vi "Init Hardware.vi"(8 "error in (no error)":errorcluster, 11 "Keithley in":refnum<class "Keithley Driver.lvclass">) -> (0 "error out":errorcluster, 3 "Keithley out":refnum<class "Keithley Driver.lvclass">)   [LabVIEW 2016, in "Keithley Driver.lvclass"]
uses:
  Keithley Driver.lvclass
  C:/github/NHMFL_Core/Libraries/Instruments/Instrument Driver/Instrument Driver.lvclass
  C:/github/NHMFL_Core/Libraries/Instruments/VISA Instrument/VISA Instrument.lvclass
  Instrument Driver/Instrument Driver.lvclass/Instrument Driver.ctl
  VISA Instrument/VISA Instrument.lvclass/VISA Instrument.ctl
  Instrument Driver/Read Recorder name.vi
  VISA Instrument/Read VISA resource.vi
  Instrument Driver/Write Channel names.vi
  Instrument Driver/Write Channel units.vi
  VISA Instrument/Write VISA resource.vi
  Read Keithley user configuration.vi
  GPIB/VISA  Send Receive.vi
  Simple VISA Reader/Simple VISA Reader Driver.lvclass
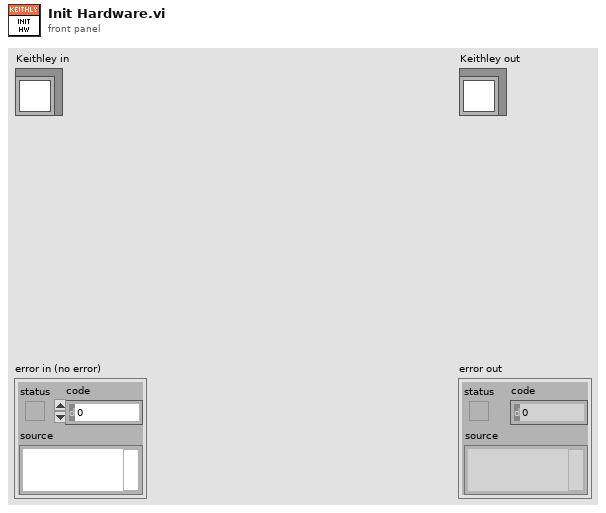
[diagram p1: front panel]
types:
  T1 = typedef "Keithley Meter Parameters.ctl" = cluster{"Range (-1: auto)":dbl, "Integration Time (NPLCs)":dbl, "Function":T2, "W Offset comp":bool, "4-wire W":bool, "Scale":dbl, "Offset":dbl}
  T2 = typedef "KeithleyMeter Function.ctl" = enum16{"VOLTAGE", "CURRENT", "RESISTANCE"}
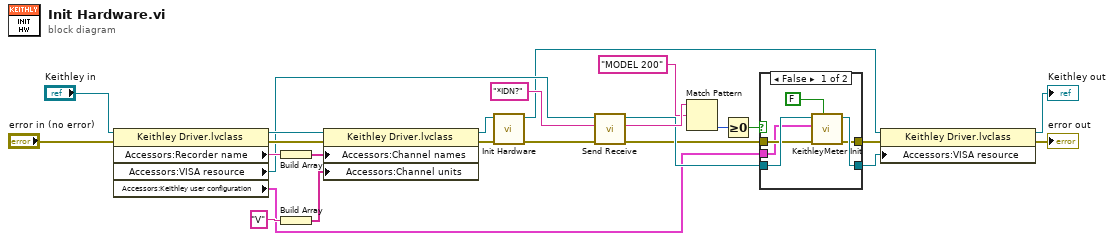
[diagram p0: block diagram]
diagram:
  n1 = property class="Keithley Driver.lvclass"(reference="Keithley in", error in="error in (no error)") -> (reference out=w22:refnum<class "Keithley Driver.lvclass">, error out=w21:errorcluster, "Accessors:Recorder name"=w20:string, "Accessors:VISA resource"=w15:refnum<visa-resource-name>, "Accessors:Keithley user configuration"=w4:T1)
  n2 = Build Array(w20) -> (w25:string[])
  n3 = Build Array("V") -> (w23:string[])
  n4 = property class="Keithley Driver.lvclass"(reference=w22, error in=w21, "Accessors:Channel names"=w25, "Accessors:Channel units"=w23) -> (reference out=w16:refnum<class "Keithley Driver.lvclass">, error out=w18:errorcluster)
  n5 = call-parent "Init Hardware.vi"("error in (no error)"=w18, "Instrument Driver in"=w16) -> ("error out"=w8:errorcluster, "Instrument Driver out"=w3:refnum<class "Keithley Driver.lvclass">)  [unwired: 8 in]
  n6 = call-poly "Send Receive.vi"("error in (no error)"=w8, "data string in"="*IDN?", "VISA Resource Name"=w15) -> ("error out"=w7:errorcluster, "data string out"=w13:string, "VISA Resource Name Out"=w9:refnum<visa-resource-name>)  [unwired: 6 in]
  n7 = Match Pattern(string=w13, regular expression="MODEL 200") -> (offset past match=w11:i32)  [unwired: 1 in, 3 out]
  n8 = Greater Or Equal To 0?(x=w11) -> (x >= 0?=w10:bool)
  n9 = case shown="False" w10 {
    tunnel: w9 -> [w31 w33]
    tunnel: w7 -> [w30 w32]
    tunnel: [w29 w33] -> w6
    tunnel: [w28 w32] -> w5
    tunnel: w4 -> [w27 _]
    frame False {
      n10 = call "KeithleyMeter Init.vi"("Source-meter"=FALSE, "Error In"=w30, "Parameters"=w27, "VISA resource name"=w31) -> ("Error Out"=w28:errorcluster, "VISA resource name out"=w29:refnum<visa-resource-name>)  [unwired: 6 in]
    }
    frame True {
    }
  }
  n11 = property class="Keithley Driver.lvclass"(reference=w3, error in=w5, "Accessors:VISA resource"=w6) -> (reference out=→"Keithley out":refnum<class "Keithley Driver.lvclass">, error out=→"error out":errorcluster)
